vi "SIGLENT_SPD3303X-E__VISA__IDN_v00.vi"() -> ()   [LabVIEW 2020]
uses:
  controls/SCPI_enum.ctl
  variables/varSCPI.vi
panel:
  in  "SCIPI":T1 items=["*IDN?", "*SAV 1", "*RCL 1", "INSTrument CH1", "INSTrument CH2", "INSTrument?", "MEASure:CURRent? CH1", "MEASure:CURRent? CH2", "MEASure:VOLTage? CH1", "MEASure:VOLTage? CH2", "MEASure:POWEr? CH1", "MEASure:POWEr? CH2", "CH1:CURRent? ", ""]
  in  "stop":bool
  out "read buffer":string
  out "error out":errorcluster
  in  "VISA resource name":refnum<visa-resource-name>
  in  "RUN":bool
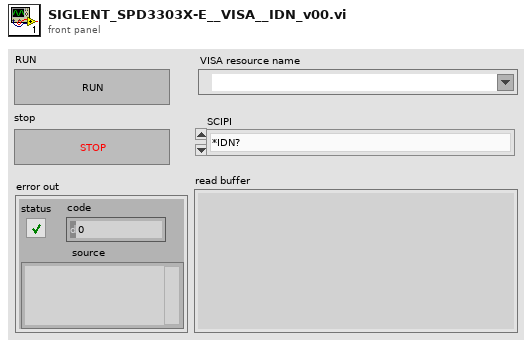
[diagram p1: front panel]
types:
  T1 = typedef "SCPI_enum.ctl" = u16
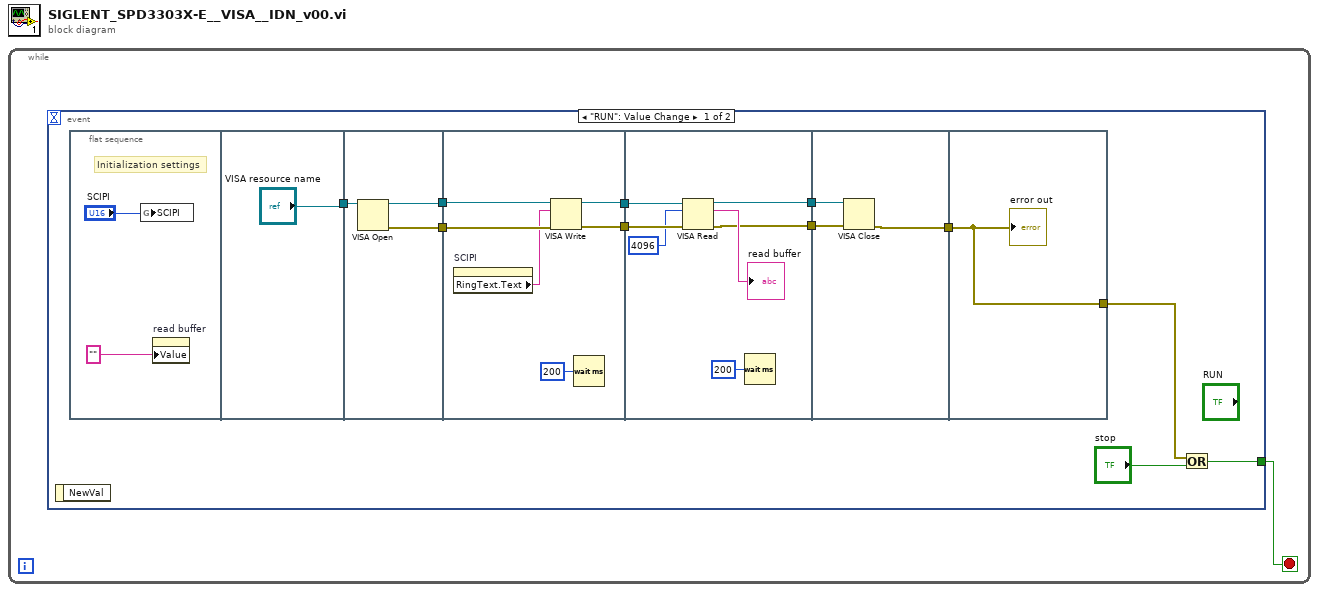
[diagram p0: block diagram]
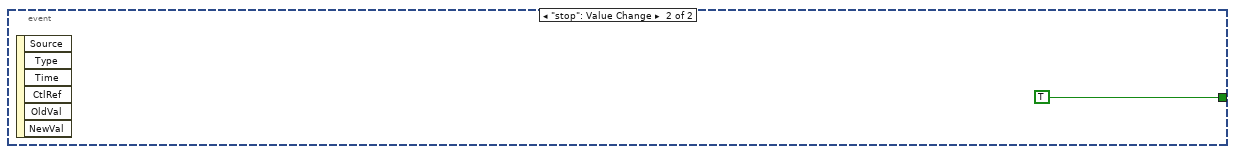
[diagram p2: hidden frame]
diagram:
  n1 = while {
    stop <- w1 stop-if-true
    n2 = event shown="[0] \"RUN\": Value Change" {
      selector: _ -> [_ _]
      dyn-events: _ -> [_ _]
      timeout: _ -> [_ _]
      tunnel: [w12 TRUE ("stop")] -> w1
      event "RUN": Value Change {
        n3 = event-data() -> ()  [unwired: 1 in, 1 out]
        n4 = flat-sequence {
          tunnel: ["VISA resource name"] -> w10
          tunnel: w10 -> [w18]
          tunnel: [w17] -> w9
          tunnel: [w16] -> w8
          tunnel: w9 -> [w24]
          tunnel: w8 -> [w23]
          tunnel: [w22] -> w7
          tunnel: [w21] -> w6
          tunnel: w7 -> [w30]
          tunnel: w6 -> [w28]
          tunnel: [w27] -> w5
          tunnel: [w26] -> w4
          tunnel: w5 -> [w34]
          tunnel: w4 -> [w33]
          tunnel: [w32] -> w3
          tunnel: w3 -> [w35]
          tunnel: [w35] -> w2
          frame #0 {
            # "Initialization settings"
            n5 = global write "varSCPI.vi" "SCIPI"("SCIPI") -> ()
            n6 = property on="read buffer" class="Str"("Value"="" ("read buffer")) -> ()  [unwired: 2 in, 2 out]
          }
          frame #1 {
          }
          frame #2 {
            n7 = VISA Open(VISA resource name=w18) -> (VISA resource name=w16:refnum<visa-resource-name>, error out=w17:errorcluster)  [unwired: 4 in]
          }
          frame #3 {
            n8 = property on="SCIPI" class="Ring (strict)"() -> ("RingText.Text"=w20:string)  [unwired: 2 in, 2 out]
            n9 = VISA Write(VISA resource name=w23, write buffer=w20, error in (no error)=w24) -> (VISA resource name out=w21:refnum<visa-resource-name>, error out=w22:errorcluster)  [unwired: 1 out]
            n10 = Wait (ms)(milliseconds to wait=u32 200) -> ()  [unwired: 1 out]
          }
          frame #4 {
            n11 = VISA Read(VISA resource name=w28, byte count=u32 4096, error in (no error)=w30) -> (VISA resource name out=w26:refnum<visa-resource-name>, read buffer=→"read buffer":string, error out=w27:errorcluster)  [unwired: 1 out]
            n12 = Wait (ms)(milliseconds to wait=u32 200) -> ()  [unwired: 1 out]
          }
          frame #5 {
            n13 = VISA Close(VISA resource name=w33, error in (no error)=w34) -> (error out=w32:errorcluster)
          }
          frame #6 {
            "error out" <- w35
          }
        }
        n14 = Or(x=w2, y="stop") -> (x .or. y?=w12:bool)
      }
      event "stop": Value Change {
        n15 = event-data() -> ()  [unwired: 1 in, 6 out]
      }
    }
  }
